vi "ClearColumnOf2DListCtrl.vi"(10 "column":u16, 11 "ArrayRef in":refnum<vi>) -> (3 "ArrayRef out":refnum<vi>)   [LabVIEW 2018, in "Library-Ctrl.lvlib"]
uses:
  Library-Ctrl.lvlib
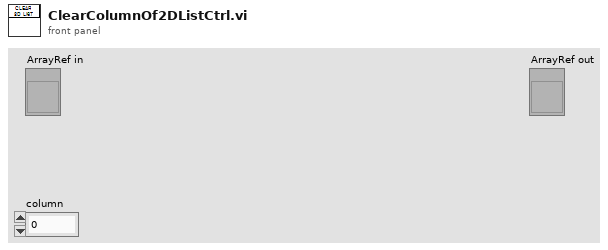
[diagram p1: front panel]
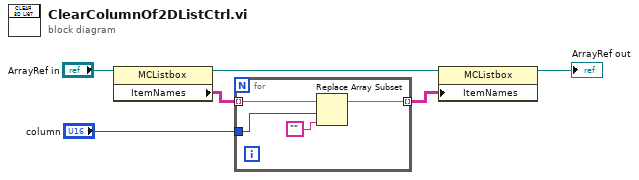
[diagram p0: block diagram]
diagram:
  n1 = property class="MCListbox"(reference="ArrayRef in") -> (reference out=w5:refnum<vi>, "ItemNames"=w6:string[][])  [unwired: 1 in, 1 out]
  n2 = for {
    tunnel: w6 -> [w10] mode=indexing
    tunnel: [w8] -> w4 mode=indexing
    tunnel: "column" -> [w7]
    n3 = Replace Array Subset(array=w10, new element="", index=w7) -> (w8:string[])
  }
  n4 = property class="MCListbox"(reference=w5, "ItemNames"=w4) -> (reference out=→"ArrayRef out":refnum<vi>)  [unwired: 1 in, 1 out]
